vi "Binarizer.vi"(8 "error in (no error)":errorcluster caption="entrée d'erreur (pas d'erreur)", 11 "Binarizer":cluster{"threshold":dbl, "copy":bool}={"threshold"=0.0, "copy"=TRUE}) -> (0 "error out":errorcluster, 3 "Binarizer en sortie":refnum<class "Binarizer.lvclass">)   [LabVIEW 2020]
doc: "Binarize data (set feature values to 0 or 1) according to a threshold\n\nValues greater than the threshold map to 1, while values less than or equal to the threshold map to 0. With the default threshold of 0, only positive values map to 1.\n\nBinarization is a common operation on text count data where the analyst can decide to only consider the presence or absence of a feature rather than a quantified number of occurrences for instance.\n\nIt can also be used as a pre-processing step for estimators that consider boolean random variables (e.g. modelled using the Bernoulli distribution in a Bayesian setting).\n\n\nParameters : \n\n- threshold : float, optional (0.0 by default)\nFeature values below or equal to this are replaced by 0, above it by 1. Threshold may not be less than 0 for operations on sparse matrices.\n\n- copy : boolean, optional, default True\nset to False to perform inplace binarization and avoid a copy (if the input is already a numpy array or a scipy.sparse CSR matrix).\n\n\nMethods :\n\n- Fit : Do nothing and return the estimator unchanged. This method is just there to implement the usual API and hence work in pipelines.\n\nParameters : X : array-like\n\n\n- Fit Transform : Fit to data, then transform it. Fits transformer to X and y with optional parameters fit_params and returns a transformed version of X.\n\nParameters : X : {array-like, sparse matrix, dataframe} of shape (n_samples, n_features)\n y : ndarray of shape (n_samples,), default=None\n Target values.\n\nReturns : X_new : ndarray array of shape (n_samples, n_features_new)\n Transformed array.\n\n\n- Transform : Binarize each element of X\n\nParameters : X : {array-like, sparse matrix}, shape [n_samples, n_features]\n The data to binarize, element by element. scipy.sparse matrices should be in CSR format to avoid an un-necessary copy."
uses:
  Binarizer.lvclass
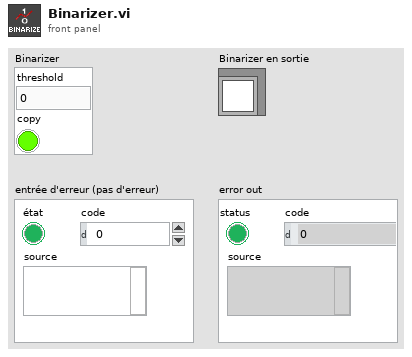
[diagram p1: front panel]
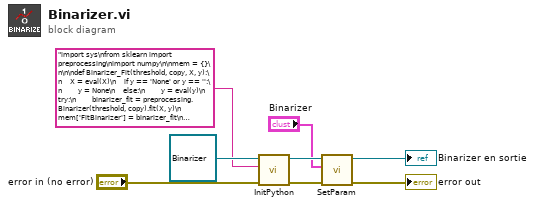
[diagram p0: block diagram]
diagram:
  n1 = call-dynamic "InitPython.vi"("error in (no error)"="error in (no error)", "Python Instruction"="import sys\nfrom sklearn import preprocessing\nimport numpy\n\nmem = {}\n\n\ndef Binarizer_Fit(threshold, copy, X, y):\n    X = eval(X)\n    if y == 'None' or y == '':\n        y = None\n    else:\n        y = eval(y)\n    try:\n        binarizer_fit = preprocessing.Binarizer(threshold, copy).fit(X, y)\n        mem['FitBinarizer'] = binarizer_fit\n        return str('OK')\n    except:\n        erreur = sys.exc_info()\n        typerr = u\"%s\" % (erreur[0])\n        typerr = typerr[typerr.find(\"'\")+1:typerr.rfind(\"'\")]\n        msgerr = u\"%s\" % (erreur[1])\n        message = str('/!\\\\ {0} : {1}'. format(typerr,msgerr))\n        return message \n    \ndef Binarizer_FitTransform(threshold, copy, X, y):\n    X = eval(X)\n    if y == 'None' or y == '':\n        y = None\n    else:\n        y = eval(y)\n    try:\n        binarizer_fit_transform = preprocessing.Binarizer(threshold, copy).fit_transform(X, y)\n        binarizer_fit_transform = binarizer_fit_transform.tolist()\n        return str(binarizer_fit_transform)\n    except:\n        erreur = sys.exc_info()\n        typerr = u\"%s\" % (erreur[0])\n        typerr = typerr[typerr.find(\"'\")+1:typerr.rfind(\"'\")]\n        msgerr = u\"%s\" % (erreur[1])\n        message = str('/!\\\\ {0} : {1}'. format(typerr,msgerr))\n        return message \n\ndef Binarizer_Transform(threshold, copy, X, y):\n    X = eval(X)\n    if y == 'None' or y == '':\n        y = None\n    else:\n        y = eval(y)\n    try:\n        binarizer_transform = mem['FitBinarizer'].transform(X)\n        binarizer_transform = binarizer_transform.tolist()\n        return str(binarizer_transform)\n    except:\n        erreur = sys.exc_info()\n        typerr = u\"%s\" % (erreur[0])\n        typerr = typerr[typerr.find(\"'\")+1:typerr.rfind(\"'\")]\n        msgerr = u\"%s\" % (erreur[1])\n        message = str('/!\\\\ {0} : {1}'. format(typerr,msgerr))\n        return message ", "Scikit-learn en entrée"=refnum<class "Binarizer.lvclass"> refnum ("Binarizer.lvclass")) -> ("error out"=w4:errorcluster, "Scikit-learn en sortie"=w5:refnum<class "Binarizer.lvclass">)  [unwired: 7 in]
  n2 = call-dynamic "SetParam.vi"("error in (no error)"=w4, "Binarizer"="Binarizer", "Binarizer en entrée"=w5) -> ("error out"=→"error out":errorcluster, "Binarizer en sortie"=→"Binarizer en sortie":refnum<class "Binarizer.lvclass">)  [unwired: 7 in]
